vi "VI-Create Typedef From Terminal.vi"(0 "Terminal":refnum<vi>, 11 "error in (no error)":errorcluster) -> (4 "typedef path":path, 15 "error out":errorcluster)   [LabVIEW 2015]
uses:
  <vilib>/Utility/miscctls.llb/LVPositionTypeDef.ctl
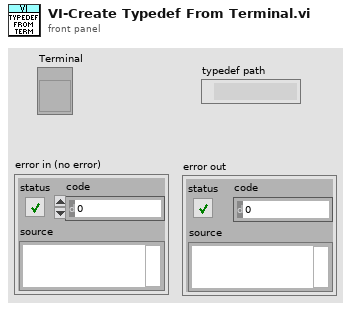
[diagram p1: front panel]
types:
  T1 = typedef "LVPositionTypeDef.ctl" = cluster{"Left":i32, "Top":i32}
  T2 = enum32{"invalid VI type", "Standard VI", "Control VI", "Global VI", "Polymorphic VI", "Configuration VI", "SubSystem", "Facade VI", "Method VI", "Statechart Diagram VI"}
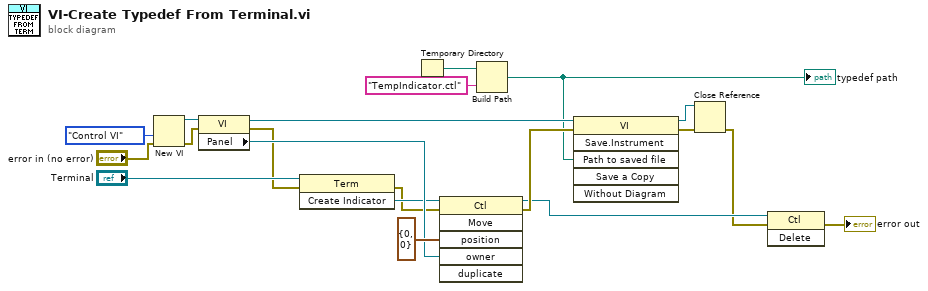
[diagram p0: block diagram]
diagram:
  n1 = New VI(8:"error in (no error)", 9:T2."Control VI" ("vi type (standard vi)")) -> (0:w13:errorcluster, 3:w18:refnum<vi>)  [unwired: 5 in]
  n2 = property class="VI"(reference=w18, error in=w13) -> (reference out=w9:refnum<vi>, error out=w12:errorcluster, "Panel"=w19:refnum<vi>)
  n3 = invoke class="Term" method="Create Indicator"(reference="Terminal", error in=w12) -> (error out=w11:errorcluster, "Create Indicator"=w17:refnum<vi>)  [unwired: 1 in, 1 out]
  n4 = Temporary Directory() -> (w1:path)
  n5 = invoke class="Ctl" method="Move"(reference=w17, error in=w11, "position"=T1 {"Left"=0, "Top"=0}, "owner"=w19) -> (reference out=w4:refnum<vi>, error out=w10:errorcluster)  [unwired: 2 in, 4 out]
  n6 = Build Path(base path=w1, name or relative path="TempIndicator.ctl") -> (appended path=w5:path)
  "typedef path" <- w5
  n7 = invoke class="VI" method="Save.Instrument"(reference=w9, error in=w10, "Path to saved file"=w5) -> (reference out=w7:refnum<vi>, error out=w8:errorcluster)  [unwired: 3 in, 4 out]
  n8 = Close Reference(reference=w7, error in (no error)=w8) -> (error out=w3:errorcluster)
  n9 = invoke class="Ctl" method="Delete"(reference=w4, error in=w3) -> (error out=→"error out":errorcluster)  [unwired: 1 in, 2 out]
